vi "Read Configuration Variant.vi"(8 "error in":errorcluster, 11 "JSON file path in":path) -> (0 "error out":errorcluster, 3 "JSON variant out":variant)   [LabVIEW 2019, in "ZenGage v3.0 UI.lvclass"]
uses:
  ZenGage v3.0 UI.lvclass
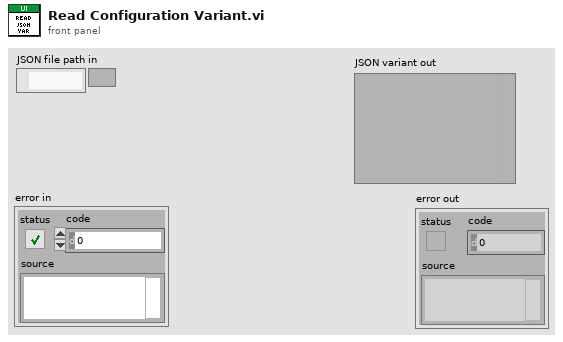
[diagram p1: front panel]
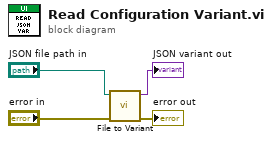
[diagram p0: block diagram]
diagram:
  n1 = call <vilib>:"File to Variant.vi"("JSON FilePath"="JSON file path in", "error in (no error)"="error in") -> ("JSON Variant"=→"JSON variant out":variant, "error out"=→"error out":errorcluster)  [unwired: 6 in, 1 out]
